vi "HW_qx_DAQ.vi"(8 "error in":errorcluster caption="错误输入") -> (0 "error out":errorcluster caption="错误输出")   [LabVIEW 2016]
uses:
  Ctrls/Read and Write Ring.ctl
  Ctrls/HardWare _ Data Queue Manage FGV Operation.ctl
  QX DAQ FGV Operations.ctl
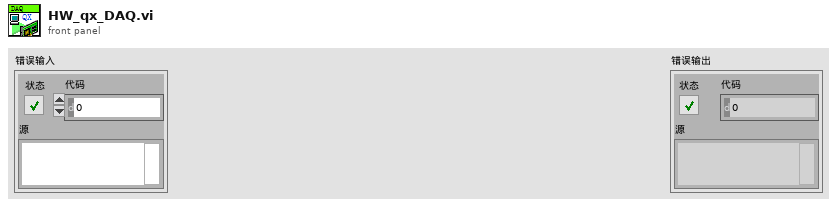
[diagram p1: front panel]
types:
  T1 = typedef "QX DAQ FGV Operations.ctl" = enum16{"Search", "ReadCFG", "UpdateTempCFG", "DownloadCFG", "StartDAQ", "RunDAQ", "StopDAQ", "DisConnect"}
  T2 = typedef "HardWare _ Data Queue Manage FGV Operation.ctl" = enum16{"Initialize", "Add Chan", "Read Chan"}
  T3 = typedef "Read and Write Ring.ctl" = enum16{"Read", "Write"}
  T4 = cluster{"queue name":string, "ChanPara.CHName":string[]}
  T5 = cluster{i32, "data":dbl[][], "SampRate":dbl, dbl}
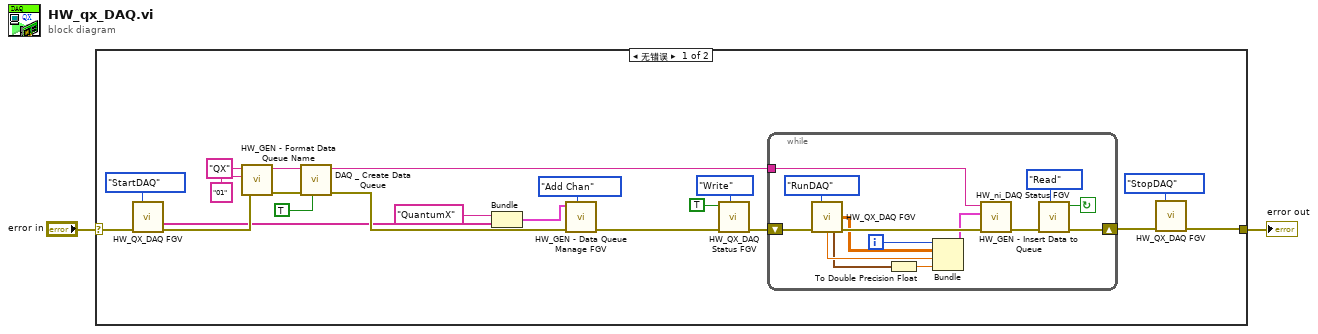
[diagram p0: block diagram]
diagram:
  n1 = case shown="无错误" "error in" {
    selector: "error in" -> [w5 w37]
    tunnel: [w7 w37] -> w1
    frame No Error {
      n2 = call "HW_QX_DAQ FGV.vi"("Oper."=QX_DAQ_FGV_Operations."StartDAQ", "error in"=w5) -> ("ChanPara.CHName"=w11:string[], "error out"=w12:errorcluster)  [unwired: 7 in, 5 out]
      n3 = call "HW_GEN - Format Data Queue Name.vi"("DevSN"="01" ("DevName"), "DevName"="QX") -> ("Q Name"=w14:string)  [unwired: 9 in]
      n4 = call "DAQ _ Create Data Queue.vi"("如未找到则创建？(T)"=TRUE, "error in"=w12, "Q-name"=w14) -> ("error out"=w18:errorcluster, "queue name"=w15:string)  [unwired: 7 in]
      n5 = Bundle("queue name"="QuantumX", "ChanPara.CHName"=w11) -> (w9:T4)  [unwired: 1 in]
      n6 = call "HW_GEN - Data Queue Manage FGV.vi"("Oper."=HardWare___Data_Queue_Manage_FGV_Operation."Add Chan", "error in"=w18, "Add Chan"=w9) -> ("error out"=w17:errorcluster)  [unwired: 7 in, 1 out]
      n7 = call "HW_QX_DAQ Status FGV.vi"("Oper"=Read_and_Write_Ring."Write", "error in"=w17, "DAQ Status in"=TRUE) -> ("error out"=w22:errorcluster)  [unwired: 7 in, 1 out]
      n8 = while {
        shift-right: [w33] -> w8
        shift-left: w22 -> [w30]
        tunnel: w15 -> [w32]
        i -> [w36]
        stop <- w34 continue-if-true
        n9 = call "HW_QX_DAQ FGV.vi"("Oper."=QX_DAQ_FGV_Operations."RunDAQ", "error in"=w30) -> ("data"=w24:dbl[][], "SampRate"=w27:dbl, "T0"=w26:timestamp, "error out"=w29:errorcluster)  [unwired: 7 in, 3 out]
        n10 = To Double Precision Float(number=w26) -> (double precision float=w25:dbl)
        n11 = Bundle(w36, "data"=w24, "SampRate"=w27, w25) -> (w23:T5)  [unwired: 1 in]
        n12 = call "HW_GEN - Insert Data to Queue.vi"("error in"=w29, "data"=w23, "Object Name"=w32) -> ("error out"=w31:errorcluster)  [unwired: 7 in, 1 out]
        n13 = call "HW_ni_DAQ Status FGV.vi"("Oper"=Read_and_Write_Ring."Read", "error in"=w31) -> ("error out"=w33:errorcluster, "DAQ Status out"=w34:bool)  [unwired: 8 in]
      }
      n14 = call "HW_QX_DAQ FGV.vi"("Oper."=QX_DAQ_FGV_Operations."StopDAQ", "error in"=w8) -> ("error out"=w7:errorcluster)  [unwired: 7 in, 6 out]
    }
    frame Error {
    }
  }
  "error out" <- w1
